vi "CreateNewGameBoard.vi"(8 "error in (no error)":errorcluster, 9 "Board Type (Open)":T4, 10 "Size":i32, 11 "Game Data in":T1) -> (0 "error out":errorcluster, 3 "Game Data out":T1)   [LabVIEW 2020]
doc: "Generates a new board and places the snake in the starting position"
uses:
  TypeDef/board-type.ctl
  TypeDef/game-data.ctl
  TypeDef/tiles-key.ctl
  TypeDef/direction.ctl
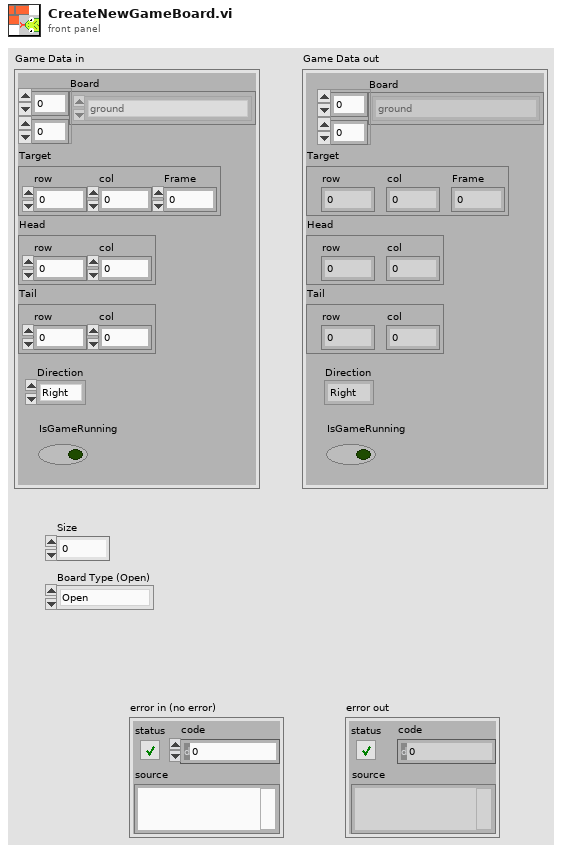
[diagram p1: front panel]
types:
  T1 = typedef "game-data.ctl" = cluster{"Board":T2[][], "Target":cluster{"row":i32, "col":i32, "Frame":i8}, "Head":cluster{"row":i32, "col":i32}, "Tail":cluster{"row":i32, "col":i32}, "Direction":T3, "IsGameRunning":bool}
  T2 = typedef "tiles-key.ctl" = enum16{"ground", "wall", "head (right)", "head (up)", "head (left)", "head (down)", "L-turn (right-up)", "L-turn (up-left)", "L-turn (left-down)", "L-turn (down-right)", "body (right)", "body (up)", "body (left)", "body (down)", "R-turn (right-down)", "R-turn (up-right)", "R-turn (left-up)", "R-turn (down-left)", "tail (right)", "tail (up)", "tail (left)", "tail (down)", "dead head (right)", "dead head (up)", "dead head (left)", "dead head (down)", "dead L-turn (right-up)", "dead L-turn (up-left)", "dead L-turn (left-down)", "dead L-turn (down-right)", "dead body (right)", "dead body (up)", "dead body (left)", "dead body (down)", "dead R-turn (right-down)", "dead R-turn (up-right)", "dead R-turn (left-up)", "dead R-turn (down-left)", "dead tail (right)", "dead tail (up)", "dead tail (left)", "dead tail (down)", "target red", "target blue", "target yellow", "target green"}
  T3 = typedef "direction.ctl" = enum16{"Right", "Up", "Left", "Down"}
  T4 = typedef "board-type.ctl" = enum16{"Open", "Fully Walled", "Walled Corners", "Cross"}
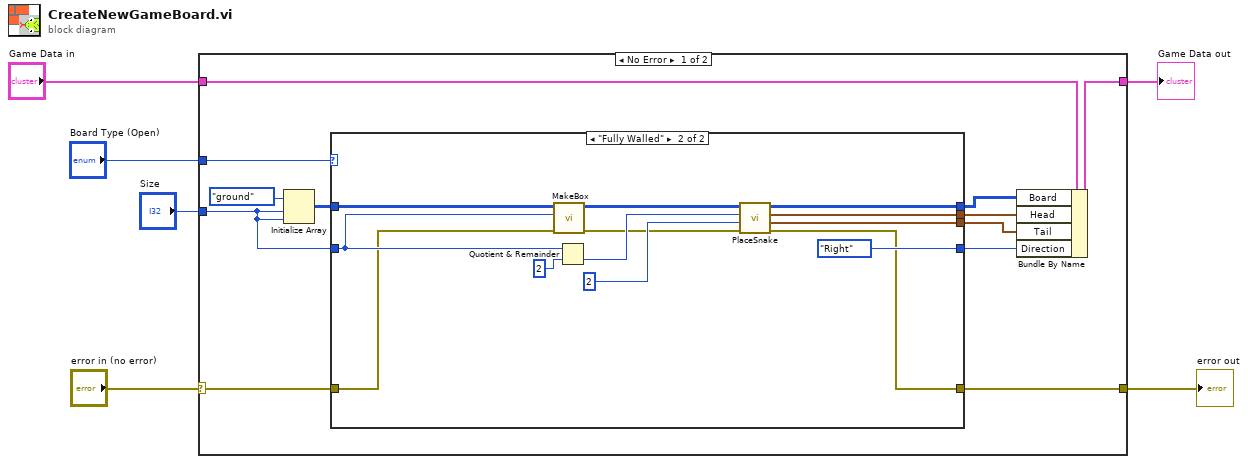
[diagram p0: block diagram]
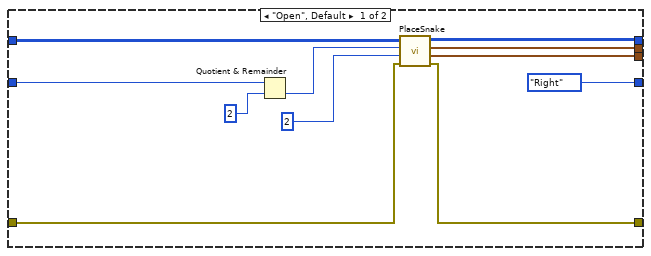
[diagram p2: hidden frame]
diagram:
  n1 = case shown="No Error" "error in (no error)" {
    selector: "error in (no error)" -> [w8 w44]
    tunnel: [w7 w44] -> w5
    tunnel: "Board Type (Open)" -> [w18 _]
    tunnel: "Size" -> [w15 _]
    tunnel: "Game Data in" -> [w10 w43]
    tunnel: [w14 w43] -> w1
    frame No Error {
      n2 = Initialize Array(tiles-key."ground" ("Tiles-key"), w15, w15) -> (w16:T2[][])
      n3 = case shown="\"Fully Walled\"" w18 {
        tunnel: w16 -> [w28 w42]
        tunnel: [w29 w40] -> w13
        tunnel: w15 -> [w24 w33]
        tunnel: [w27 w39] -> w12
        tunnel: [w26 w38] -> w11
        tunnel: [direction."Right" ("Direction") direction."Right" ("Direction")] -> w9
        tunnel: w8 -> [w20 w31]
        tunnel: [w19 w30] -> w7
        frame "Open", Default {
          n4 = Quotient & Remainder(x=w24, y=2) -> (floor(x/y)=w23:i32)  [unwired: 1 out]
          n5 = call "PlaceSnake.vi"("error in (no error)"=w20, "Tail col"=2 ("disabled index (col)"), "Tail row"=w23, "Board in"=w28) -> ("error out"=w19:errorcluster, "Tail Position"=w26:cluster{"row":i32, "col":i32}, "Head Position"=w27:cluster{"row":i32, "col":i32}, "Board out"=w29:T2[][])  [unwired: 4 in]
        }
        frame "Fully Walled" {
          n6 = call "MakeBox.vi"("error in (no error)"=w31, "Size"=w33, "Array in"=w42) -> ("error out"=w32:errorcluster, "Array out"=w41:T2[][])  [unwired: 7 in]
          n7 = Quotient & Remainder(x=w33, y=2) -> (floor(x/y)=w35:i32)  [unwired: 1 out]
          n8 = call "PlaceSnake.vi"("error in (no error)"=w32, "Tail col"=2 ("disabled index (col)"), "Tail row"=w35, "Board in"=w41) -> ("error out"=w30:errorcluster, "Tail Position"=w38:cluster{"row":i32, "col":i32}, "Head Position"=w39:cluster{"row":i32, "col":i32}, "Board out"=w40:T2[][])  [unwired: 4 in]
        }
      }
      n9 = Bundle By Name(cluster=w10, "Board"=w13, "Head"=w12, "Tail"=w11, "Direction"=w9) -> (w14:T1)
    }
    frame Error {
    }
  }
  "error out" <- w5
  "Game Data out" <- w1
